vi "GFG_Examples.vi"() -> ()   [LabVIEW 2012]
uses:
  <vilib>/Utility/VariantDataType/Type.ctl
  GFGbooleanGet.vi
  <vilib>/Utility/VariantDataType/VariantType.lvlib
  GFG library.lvlib
panel:
  in  "posX":dbl
  out "Boolean":bool
  out "moveZabs":dbl
  out "moveYabs":dbl
  out "moveXabs":dbl
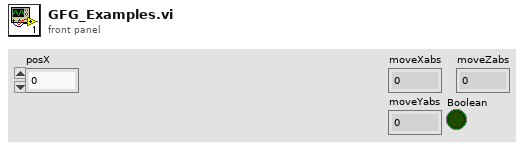
[diagram p1: front panel]
types:
  T1 = cluster{"moveXabs":dbl, "moveYabs":dbl, "moveZabs":dbl}
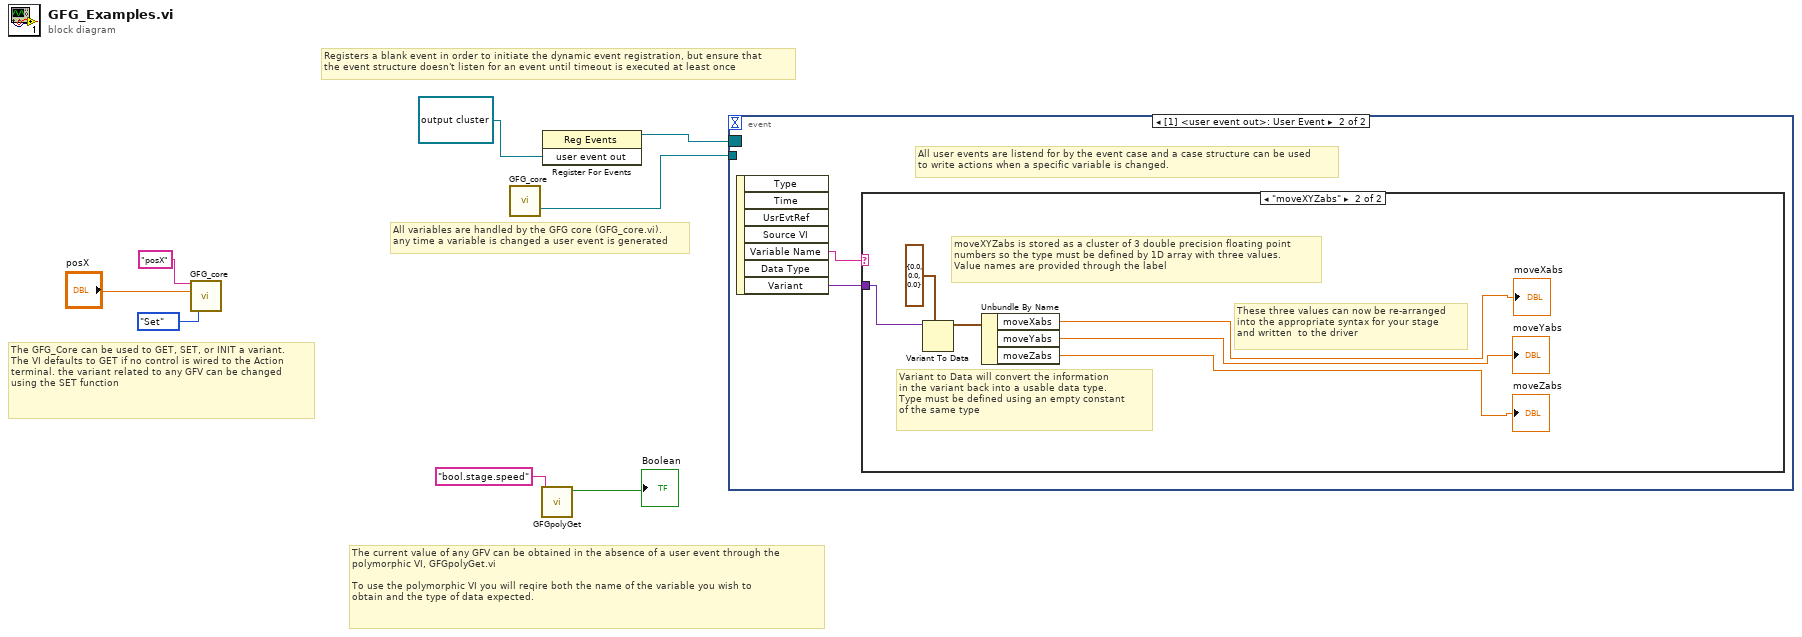
[diagram p0: block diagram]
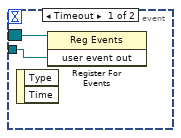
[diagram p2: hidden frame]
diagram:
  # "The GFG_Core can be used to GET, SET, or INIT a variant. \nThe VI defaults to GET if no control is wired to the Action \nterminal. the variant related to any GFV can be changed\nusing the SET function"
  # "All variables are handled by the GFG core (GFG_core.vi).\nany time a variable is changed a user event is generated"
  # "The current value of any GFV can be obtained in the absence of a user event through the polymorphic VI, GFGpolyGet.vi\n\nTo use the polymorphic VI you will reqire both the name of the variable you wish to\nobtain and the type of data expected."
  # "Registers a blank event in order to initiate the dynamic event registration, but ensure that \nthe event structure doesn't listen for an event until timeout is executed at least once"
  n1 = call "GFG_core.vi"("Variable Name in"="posX", "Variant in"="posX", "Action"=enum16{"Init", "Set", "Get"}."Set") -> ()  [unwired: 10 in, 7 out]
  n2 = call "GFG_core.vi"() -> ("user event out"=w8:refnum<user-event>)  [unwired: 13 in, 6 out]
  n3 = call-poly "GFGpolyGet.vi"("Variable Name in"="bool.stage.speed") -> ("Boolean"=→"Boolean":bool)  [unwired: 10 in]
  n4 = register-events(refnum<user-event> refnum ("user event out")) -> (reference out=w7:refnum<event-registration>)  [unwired: 2 in, 1 out]
  n5 = event shown="[1] <user event out>: User Event" {
    selector: w7 -> [w10 _]
    dyn-events: _ -> [_ _]
    timeout: _ -> [_ _]
    tunnel: w8 -> [w9 _]
    event Timeout {
      n6 = event-data() -> ()  [unwired: 1 in, 2 out]
      n7 = register-events(reference=w10, w9) -> ()  [unwired: 1 in, 2 out]
    }
    event User Event {
      # "All user events are listend for by the event case and a case structure can be used\nto write actions when a specific variable is changed."
      n8 = event-data() -> ("Variable Name"=w12:string, "Variant"=w11:variant)  [unwired: 1 in, 5 out]
      n9 = case shown="\"moveXYZabs\"" w12 {
        tunnel: w11 -> [_ w18]
        frame "False", Default {
        }
        frame "moveXYZabs" {
          # "These three values can now be re-arranged \ninto the appropriate syntax for your stage  \nand written  to the driver"
          # "moveXYZabs is stored as a cluster of 3 double precision floating point\nnumbers so the type must be defined by 1D array with three values. \nValue names are provided through the label"
          # "Variant to Data will convert the information\nin the variant back into a usable data type. \nType must be defined using an empty constant \nof the same type"
          n10 = Variant To Data(type=T1 {"moveXabs"=0.0, "moveYabs"=0.0, "moveZabs"=0.0} ("output cluster"), Variant=w18) -> (data=w16:T1)  [unwired: 1 in, 1 out]
          n11 = Unbundle By Name(w16) -> ("moveXabs"=→"moveXabs":dbl, "moveYabs"=→"moveYabs":dbl, "moveZabs"=→"moveZabs":dbl)
        }
      }
    }
  }
